vi "New NetCPU.vi"(8 "instVIpath":path, 9 "target location":string, 11 "NetCPU in":refnum<class "NetCPU.lvclass">) -> (3 "NetCPU out":refnum<class "NetCPU.lvclass">)   [LabVIEW 2020, in "NI_TargetHelper.lvlib" / "NetCPU.lvclass"]
uses:
  <vilib>/TargetSupport/NI_TargetHelper/NetCPU/NetCPU.lvclass
  <vilib>/TargetSupport/NI_TargetHelper/NetCPU/NetCPU.lvclass/NetCPU.ctl
  <vilib>/TargetSupport/NI_TargetHelper/NI_TargetHelper.lvlib
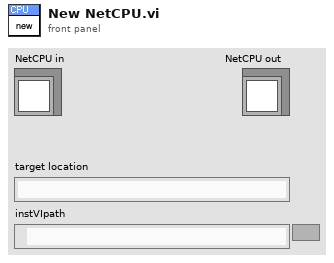
[diagram p1: front panel]
types:
  T1 = typedef "NI_TargetHelper.lvlib/Instance VIref.ctl" = refnum<vi>
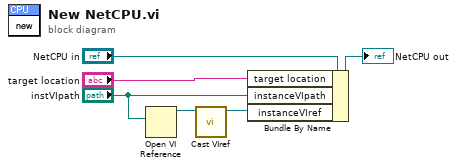
[diagram p0: block diagram]
diagram:
  n1 = Open VI Reference(vi path="instVIpath") -> (vi reference=w2:refnum<vi>)  [unwired: 5 in, 1 out]
  n2 = call <vilib>:"Cast VIref.vi"("VI Refnum"=w2) -> ("instVIref"=w1:T1)  [unwired: 10 in]
  n3 = Bundle By Name(cluster="NetCPU in", "target location"="target location", "instanceVIpath"="instVIpath", "instanceVIref"=w1) -> (→"NetCPU out":refnum<class "NetCPU.lvclass">)
